vi "GetDataForExcel.ExtractData.ReadFile.vi"(9 "index":i32, 10 "relative path":string, 11 "base path":path) -> (3 "data":dbl)   [LabVIEW 2013, in "main.lvlib"]
uses:
  main.lvlib
  <userlib>/_OpenG.lib/file/file.llb/File Exists - Scalar__ogtk.vi
  <vilib>/Utility/file.llb/Read From Spreadsheet File (DBL).vi
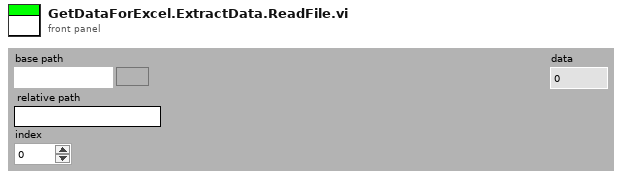
[diagram p1: front panel]
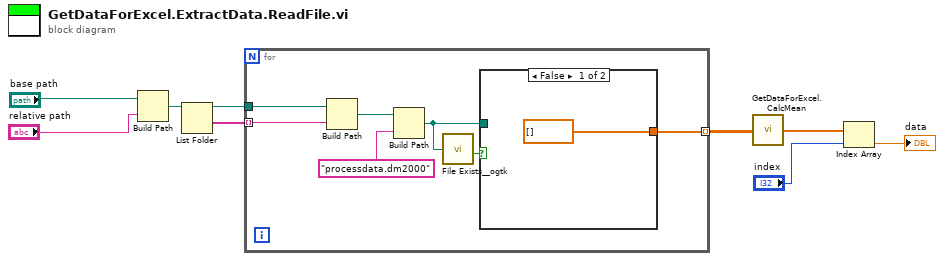
[diagram p0: block diagram]
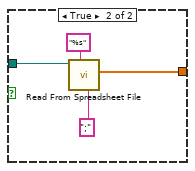
[diagram p2: hidden frame]
diagram:
  n1 = Build Path(base path="base path", name or relative path="relative path") -> (appended path=w7:path)
  n2 = List Folder(path=w7) -> (path out=w6:path, folder names=w5:string[])  [unwired: 3 in, 2 out]
  n3 = for {
    tunnel: w6 -> [w12]
    tunnel: w5 -> [w11] mode=indexing
    tunnel: [w10] -> w4 mode=indexing
    n4 = Build Path(base path=w12, name or relative path=w11) -> (appended path=w14:path)
    n5 = Build Path(base path=w14, name or relative path="processdata.dm2000") -> (appended path=w16:path)
    n6 = call-poly <userlib>:"File Exists__ogtk.vi"("file path"=w16) -> ("exists"=w15:bool)  [unwired: 6 in, 1 out]
    n7 = case shown="False" w15 {
      tunnel: [dbl[] [] w19] -> w10
      tunnel: w16 -> [_ w18]
      frame False {
      }
      frame True {
        n8 = call-poly <vilib>:"Read From Spreadsheet File.vi"("delimiter (\\t)"=";" ("delimiter (\\t)"), "format (%.3f)"="%s", "file path (dialog if empty)"=w18) -> ("first row"=w19:dbl[])  [unwired: 4 in, 4 out]
      }
    }
  }
  n9 = call "GetDataForExcel.CalcMean.vi"("Input Array"=w4) -> ("Array"=w3:dbl[])
  n10 = Index Array(array=w3, index="index") -> (element=→"data":dbl)
